vi "旋轉測試.vi"() -> ()   [LabVIEW 2015]
uses:
  <vilib>/vision/driver/NI_Vision_Acquisition_Software.lvlib
  <vilib>/vision/NI_Vision_Development_Module.lvlib
panel:
  in  "Option":T1={"X個數"=6, "Y個數"=3, "起始X"=78.0, "起始Y"=60.0, "位移X"=87.0, "位移Y"=87.0, "抖動range"=0.0}
  in  "input variable":dbl
  in  "Path Array":path[](array[path])
  in  "ROI數量":i32=1
  in  "Don't need to press Ctrl To ZoomIn/ZoomOut":bool
  in  "Cameraindex":i32
  in  "持續更新":bool
  in  "使用固定圖片":bool
  in  "開圖":bool=TRUE
  in  "影像數量":i32=1
  in  "ImageIndex":i32(slide) min=0 scale=0.0..1.0
  in  "重新開圖":bool
  in  "取像":bool
  out "error out":errorcluster
  in  "stop":bool
  out "Image":T2(plugin-control)
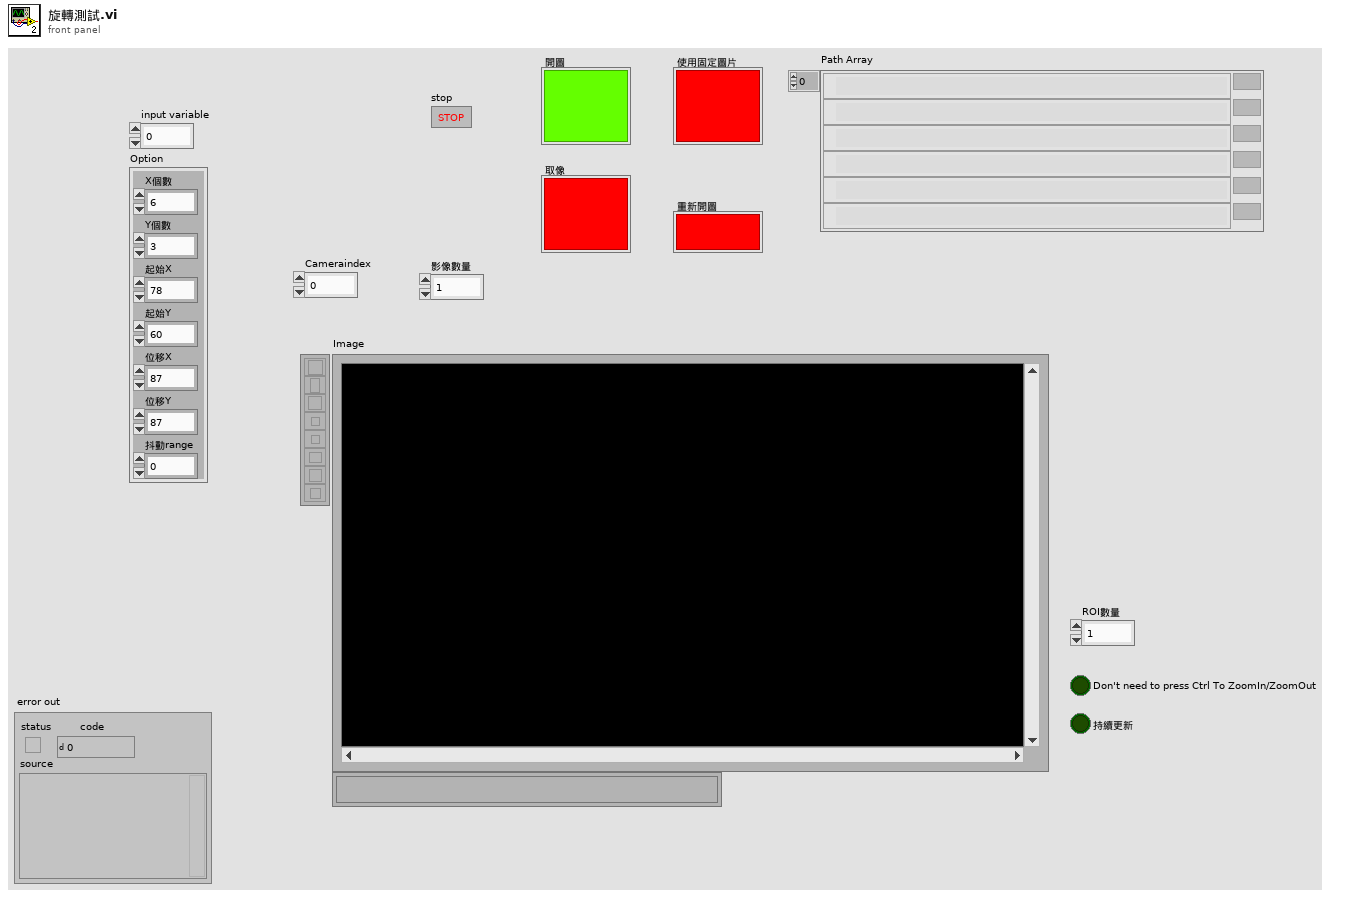
[diagram p1: front panel]
types:
  T1 = cluster{"X個數":i32, "Y個數":i32, "起始X":dbl, "起始Y":dbl, "位移X":dbl, "位移Y":dbl, "抖動range":dbl}
  T2 = typedef "IMAQ Image.ctl" = refnum<image>
  T3 = cluster{"Type":u32, "Version":u32, "Flags":u32, "SerialNumberHigh":u32, "SerialNumberLow":u32, "BusType":u32, "InterfaceName":string, "VendorName":string, "ModelName":string, "CameraFileName":string, "CameraAttributeURL":string}[]
  T4 = typedef "IMAQdx.ctl" = refnum<k21>
  T5 = cluster{"Global Rectangle":i32[], "Contours":cluster{"Contour Type":u32, "ROI Type":u32, "Points":i32[]}[]}
  T6 = cluster{"ROI":cluster{"Global Rectangle":i32[], "Contours":cluster{"Contour Type":u32, "ROI Type":u32, "Points":i32[]}[]}, "input variable":dbl, "Option":cluster{"X個數":i32, "Y個數":i32, "起始X":dbl, "起始Y":dbl, "位移X":dbl, "位移Y":dbl, "抖動range":dbl}}
  T7 = cluster{"重新開圖":bool, "取像":bool, "Cameraindex":i32, "ImageIndex":i32, cluster{"ROI":cluster{"Global Rectangle":i32[], "Contours":cluster{"Contour Type":u32, "ROI Type":u32, "Points":i32[]}[]}, "input variable":dbl, "Option":cluster{"X個數":i32, "Y個數":i32, "起始X":dbl, "起始Y":dbl, "位移X":dbl, "位移Y":dbl, "抖動range":dbl}}}
  T8 = typedef "IMAQ Point" = cluster{"X":sgl, "Y":sgl}
  T9 = typedef "Image action.ctl" = enum16{"初始化", "創造記憶體", "寫入圖片", "讀取圖片", "刪除圖片", "等待"}
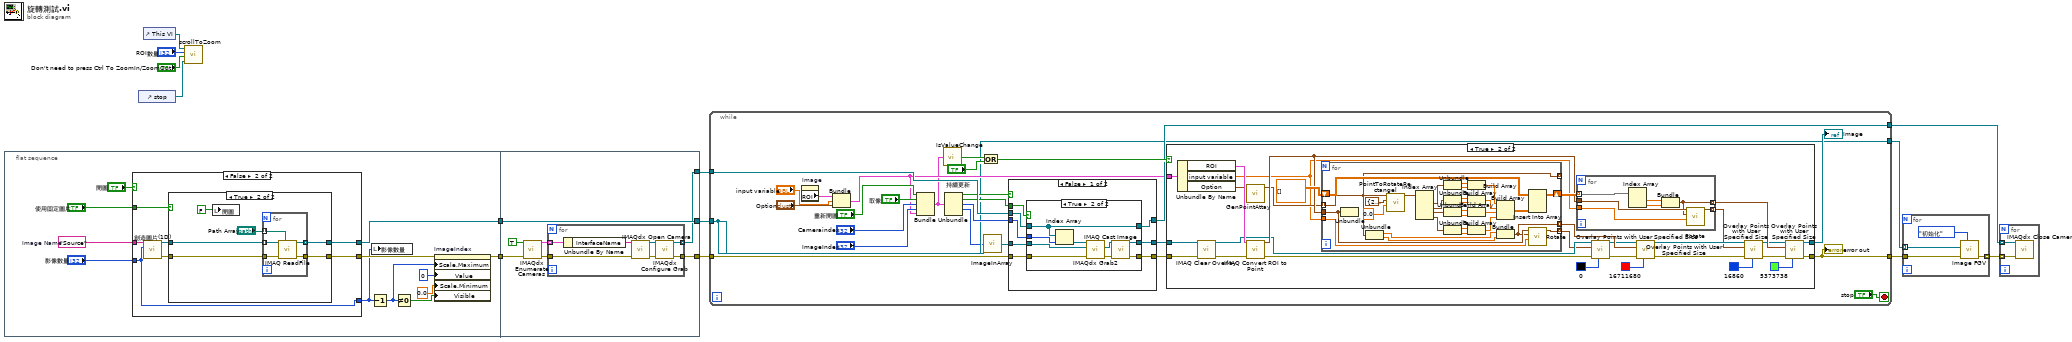
[diagram p0: block diagram]
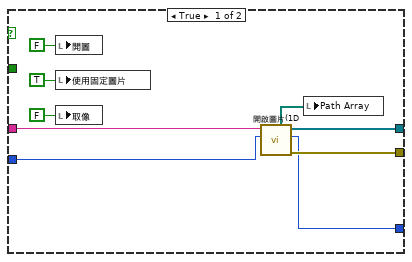
[diagram p2: hidden frame]
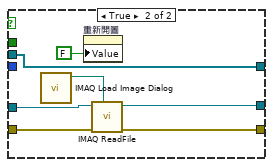
[diagram p5: hidden frame]
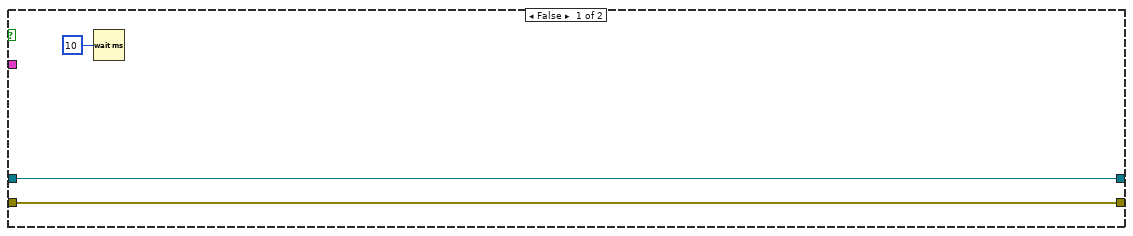
[diagram p6: hidden frame]
diagram:
  n1 = flat-sequence {
    tunnel: [w18] -> w12
    tunnel: [w25] -> w11
    tunnel: [w55] -> w10
    tunnel: [w61] -> w13
    tunnel: w12 -> [w61]
    tunnel: w11 -> [w58]
    tunnel: [w57] -> w5
    frame #0 {
      w21 = "Source"  # Image Name
      n2 = case shown="False" "開圖" {
        tunnel: w21 -> [w31 w41]
        tunnel: "影像數量" -> [w30 w35]
        tunnel: [w29 w38] -> w19
        tunnel: [w28 w39] -> w18
        tunnel: [w27 w35] -> w14
        tunnel: "使用固定圖片" -> [_ w36]
        frame True {
          n3 = local write "開圖"(FALSE ("取像")) -> ()
          n4 = local write "使用固定圖片"(TRUE ("取像")) -> ()
          n5 = local write "取像"(FALSE ("取像")) -> ()
          n6 = call "開啟圖片(1D.vi"("影像數量"=w30, "Image Name"=w31) -> ("error out"=w29:errorcluster, "ImagePathNumber"=w27:i32, "Image1DArray"=w28:T2[], "ImagePath"=w26:path[])  [unwired: 5 in, 1 out]
          n7 = local write "Path Array"(w26) -> ()
        }
        frame False {
          n8 = call "創造圖片(1D).vi"("影像數量"=w35, "Image Name"=w41) -> ("error out"=w37:errorcluster, "Image1DArray"=w40:T2[])  [unwired: 7 in, 1 out]
          n9 = case shown="True" w36 {
            tunnel: w40 -> [w42 w49]
            tunnel: [w42 w44] -> w39
            tunnel: [w43 w47] -> w38
            tunnel: w37 -> [w43 w46]
            frame False {
            }
            frame True {
              n10 = local write "開圖"(FALSE ("取像")) -> ()
              n11 = for {
                tunnel: w49 -> [w50] mode=indexing
                tunnel: "Path Array" -> [w54] mode=indexing
                tunnel: [w53] -> w44 mode=indexing
                tunnel: w46 -> [w51]
                tunnel: [w52] -> w47
                n12 = call "IMAQ ReadFile"("File Path"=w54, "error in (no error)"=w51, "Image"=w50) -> ("error out"=w52:errorcluster, "Image Out"=w53:T2)  [unwired: 4 in, 3 out]
              }
            }
          }
        }
      }
      n13 = Decrement(x=w14) -> (x-1=w23:i32)
      n14 = local write "影像數量"(w14) -> ()
      n15 = Not Equal To 0?(x=w23) -> (x != 0?=w22:bool)
      n16 = property on="ImageIndex" class="Slide (strict)"(error in=w19, "Scale.Maximum"=w23, "Value"=0 ("Scale.Range:Minimum"), "Scale.Minimum"=0.0 ("Scale.Range:Minimum"), "Visible"=w22) -> (error out=w25:errorcluster)  [unwired: 1 in, 1 out]
    }
    frame #1 {
      n17 = call <vilib>:"IMAQdx Enumerate Cameras.vi"("error in"=w58, "Connected Only? (Yes)"=TRUE ("Connected Only?")) -> ("error out"=w56:errorcluster, "Camera Information Array"=w59:T3)  [unwired: 8 out]
      n18 = for {
        tunnel: w59 -> [w68] mode=indexing
        tunnel: [w64] -> w57 mode=indexing
        tunnel: w56 -> [w66]
        tunnel: [w62] -> w55
        n19 = Unbundle By Name(w68) -> ("InterfaceName"=w67:string)
        n20 = call <vilib>:"IMAQdx Open Camera.vi"("error in"=w66, "Session In"=w67) -> ("error out"=w63:errorcluster, "Session Out"=w65:T4)  [unwired: 1 in, 7 out]
        n21 = call <vilib>:"IMAQdx Configure Grab.vi"("error in"=w63, "Session In"=w65) -> ("error out"=w62:errorcluster, "Session Out"=w64:T4)  [unwired: 8 out]
      }
    }
  }
  n22 = control-ref of="stop"() -> (w6:refnum<vi>)
  n23 = control-ref of="This VI"() -> (w9:refnum<vi>)
  n24 = call "scrollToZoom.vi"("stop"=w6, "Don't need to press Ctrl To ZoomIn/ZoomOut"="Don't need to press Ctrl To ZoomIn/ZoomOut", "ROI數量"="ROI數量", "VI in"=w9) -> ()  [unwired: 8 in]
  n25 = while {
    tunnel: w13 -> [w73]
    tunnel: w10 -> [w90]
    tunnel: w5 -> [w87]
    tunnel: [w79] -> w3
    tunnel: [w73] -> w2
    tunnel: [w78] -> w1
    stop <- "stop" stop-if-true
    n26 = property on="Image" class="ImageControl"() -> ("ROI"=w76:T5)  [unwired: 2 in, 2 out]
    n27 = Bundle("ROI"=w76, "input variable"="input variable", "Option"="Option") -> (w75:T6)  [unwired: 1 in]
    n28 = Bundle("重新開圖"="重新開圖", "取像"="取像", "Cameraindex"="Cameraindex", "ImageIndex"="ImageIndex", w75) -> (w74:T7)  [unwired: 1 in]
    n29 = call "IsValueChange.vi"("Variant"=w74) -> ("result"=w77:bool)
    n30 = Unbundle(w74) -> ("重新開圖"=w82:bool, "取像"=w81:bool, "Cameraindex"=w80:i32, "ImageIndex"=w71:i32)  [unwired: 1 out]
    n31 = Or(x=w77, y="持續更新") -> (x .or. y?=w91:bool)
    n32 = call "ImageInArray.vi"("index"=w71, "Array"=w73) -> ("Image"=w72:T2)
    n33 = case shown="False" w82 {
      tunnel: [w98 w121] -> w89
      tunnel: w90 -> [w102 w117]
      tunnel: [w99 w118] -> w88
      tunnel: w81 -> [w101 _]
      tunnel: [w100 w116] -> w78
      tunnel: w87 -> [w97 w116]
      tunnel: w80 -> [w96 _]
      tunnel: w72 -> [w95 w115]
      frame False {
        n34 = case shown="True" w101 {
          tunnel: [w104 w109] -> w100
          tunnel: [w103 w114] -> w98
          tunnel: w102 -> [w105 w107]
          tunnel: [w105 w110] -> w99
          tunnel: w97 -> [w104 w109]
          tunnel: w96 -> [_ w108]
          tunnel: w95 -> [w103 w106]
          frame False {
          }
          frame True {
            n35 = Index Array(array=w109, index=w108) -> (element=w111:T4)
            n36 = call <vilib>:"IMAQdx Grab2.vi"("error in"=w107, "Image In"=w106, "Session In"=w111) -> ("error out"=w112:errorcluster, "Image Out"=w113:T2)  [unwired: 5 in, 2 out]
            n37 = call "IMAQ Cast Image"("error in (no error)"=w112, "Image Src"=w113) -> ("error out"=w110:errorcluster, "Image Dst Out"=w114:T2)  [unwired: 8 in]
          }
        }
      }
      frame True {
        n38 = call "IMAQ Load Image Dialog"() -> ("Path"=w119:path)  [unwired: 9 in, 2 out]
        n39 = property on="重新開圖" class="Bool (strict)"("Value"=FALSE ("重新開圖")) -> ()  [unwired: 2 in, 2 out]
        n40 = call "IMAQ ReadFile"("File Path"=w119, "error in (no error)"=w117, "Image"=w115) -> ("error out"=w118:errorcluster, "Image Out"=w121:T2)  [unwired: 4 in, 3 out]
      }
    }
    n41 = case shown="True" w91 {
      tunnel: [w123 w147] -> w93
      tunnel: w89 -> [w123 w153]
      tunnel: w88 -> [w122 w152]
      tunnel: [w122 w148] -> w79
      tunnel: w75 -> [_ w151]
      frame False {
        n42 = Wait (ms)(milliseconds to wait=u32 10) -> ()  [unwired: 1 out]
      }
      frame True {
        n43 = Unbundle By Name(w151) -> ("ROI"=w142:T5, "input variable"=w125:dbl, "Option"=w126:T1)
        n44 = call "IMAQ Clear Overlay"("error in (no error)"=w152, "Image"=w153) -> ("error out"=w141:errorcluster, "Image Out"=w133:T2)  [unwired: 8 in]
        n45 = call <userlib>:"GenPointAttay.vi"("Option"=w126) -> ("Output Points"=w127:cluster{"X":dbl, "Y":dbl}[])  [unwired: 9 in, 1 out]
        n46 = call "IMAQ Convert ROI to Point"("error in (no error)"=w141, "ROI Descriptor"=w142) -> ("error out"=w131:errorcluster, "Point"=w134:T8)  [unwired: 7 in]
        n47 = for {
          shift-right: [w188] -> w143
          shift-left: dbl[][] [] -> [w189]
          tunnel: [w185] -> w145 mode=indexing
          tunnel: w125 -> [w187]
          tunnel: w134 -> [w186]
          tunnel: [w184] -> w129 mode=indexing
          tunnel: [w163] -> _ mode=indexing
          tunnel: w127 -> [w163] mode=indexing
          n48 = Unbundle(w186) -> ()  [unwired: 2 out]
          n49 = Unbundle(w163) -> ("X"=w162:dbl, "Y"=w161:dbl)
          n50 = call <userlib>:"PointToRotateRectangel.vi"("rotate"=0.0 ("totate"), "Size"=cluster{"Width":sgl, "Height":sgl} {"Width"=25.0, "Height"=25.0}, "Center Point"=w163) -> ("Output Points"=w179:T8[])  [unwired: 7 in, 1 out]
          n51 = Index Array(array=w179) -> (element #1=w175:T8, element #2=w176:T8, element #3=w177:T8, element #4=w178:T8)  [unwired: 4 in]
          n52 = Unbundle(w175) -> ("X"=w174:sgl, "Y"=w173:sgl)
          n53 = Unbundle(w176) -> ("X"=w172:sgl, "Y"=w171:sgl)
          n54 = Unbundle(w177) -> ("X"=w170:sgl, "Y"=w169:sgl)
          n55 = Unbundle(w178) -> ("X"=w168:sgl, "Y"=w167:sgl)
          n56 = Build Array(w174, w173) -> (w183:sgl[])
          n57 = Build Array(w172, w171) -> (w182:sgl[])
          n58 = Build Array(w170, w169) -> (w181:sgl[])
          n59 = Build Array(w168, w167) -> (w180:sgl[])
          n60 = Build Array(w183, w182, w181, w180) -> (w166:sgl[][])
          n61 = Bundle("X"=w162, "Y"=w161) -> (w185:cluster{"X":dbl, "Y":dbl})  [unwired: 1 in]
          n62 = Insert Into Array(array=w189, new element=w166) -> (w188:dbl[][])  [unwired: 2 in]
          n63 = call <userlib>:"Rotate.vi"("Rotate"=w187, "Input Point"=w185, "Rotation center Point"=w186) -> ("Output Point"=w184:cluster{"X":dbl, "Y":dbl})  [unwired: 7 in, 1 out]
        }
        n64 = for {
          tunnel: w143 -> [w160] mode=indexing
          tunnel: [w155] -> w149 mode=indexing
          tunnel: w134 -> [w156]
          tunnel: [w157] -> w135 mode=indexing
          tunnel: w125 -> [w154]
          n65 = Index Array(array=w160) -> (element #1=w159:dbl, element #2=w158:dbl)  [unwired: 2 in]
          n66 = Bundle(w159, w158) -> (w155:cluster{dbl, dbl})  [unwired: 1 in]
          n67 = call <userlib>:"Rotate.vi"("Rotate"=w154, "Input Point"=w155, "Rotation center Point"=w156) -> ("Output Point"=w157:cluster{"X":dbl, "Y":dbl})  [unwired: 7 in, 1 out]
        }
        n68 = call "Overlay Points with User Specified Size.vi"("Color"=u32 0, "error in"=w131, "Points"=w129, "Image In"=w133) -> ("error out"=w130:errorcluster, "Image Out"=w132:T2)  [unwired: 6 in]
        n69 = call "Overlay Points with User Specified Size.vi"("Color"=u32 16711680, "error in"=w130, "Points"=w145, "Image In"=w132) -> ("error out"=w140:errorcluster, "Image Out"=w138:T2)  [unwired: 6 in]
        n70 = call "Overlay Points with User Specified Size.vi"("Color"=u32 16860, "error in"=w140, "Points"=w135, "Image In"=w138) -> ("error out"=w139:errorcluster, "Image Out"=w137:T2)  [unwired: 6 in]
        n71 = call "Overlay Points with User Specified Size.vi"("Color"=u32 5373738, "error in"=w139, "Points"=w149, "Image In"=w137) -> ("error out"=w148:errorcluster, "Image Out"=w147:T2)  [unwired: 6 in]
      }
    }
    "Image" <- w93
    "error out" <- w79
  }
  n72 = for {
    tunnel: w2 -> [w193] mode=indexing
    tunnel: [w191] -> w4 mode=indexing
    tunnel: w3 -> [w190]
    n73 = call "Image FGV.vi"("Image action"=Image_action."初始化", "error in (no error)"=w190, "Image In"=w193) -> ("error out"=w191:errorcluster)  [unwired: 7 in, 1 out]
  }
  n74 = for {
    tunnel: w1 -> [w195] mode=indexing
    tunnel: w4 -> [w194] mode=indexing
    n75 = call <vilib>:"IMAQdx Close Camera.vi"("error in"=w194, "Session In"=w195) -> ()  [unwired: 9 in, 1 out]
  }
